vi "ENAmeas.vi"(4 "Error In (no error)":errorcluster, 5 "Meas":T1, 6 "ENA Config":T2={"Sweep Type"=0, "Sweep Mode"=0, "Sweep Points"=201, "Average count"=16, "IF Bandwidth (Hz)"=100000.0, "Power Level (dBm)"=0.0, "Center Freq (Hz)"=0.0, "Span Freq (Hz)"=0.0, "Electrical Delay (s)"=0.0} {"Electrical Delay (s)" format="%.2p"; "Span Freq (Hz)" format="%.2p"; "Center Freq (Hz)" format="%.2p"; "Power Level (dBm)" format="%^.2g"; "IF Bandwidth (Hz)" format="%.1p"; "Sweep Mode" items=["Stepped", "Swept", "Fast Stepped Mode", "Fast Swept Mode"]; "Sweep Type" items=["Linear Sweep", "Logarithmic Sweep", "Segment Sweep", "Power Sweep", "DC Bias"]}, 7 "VISA session":refnum<visa-resource-name>) -> (0 "Error Out":errorcluster, 1 "ENAfreq":dbl[](array[numeric]), 2 "ENAdata":dbl[][](array[numeric]), 3 "dup VISA session":refnum<visa-resource-name>)   [LabVIEW 2017]
uses:
  <instrlib>/Agilent ENA Series/Agilent ENA Series.lvlib
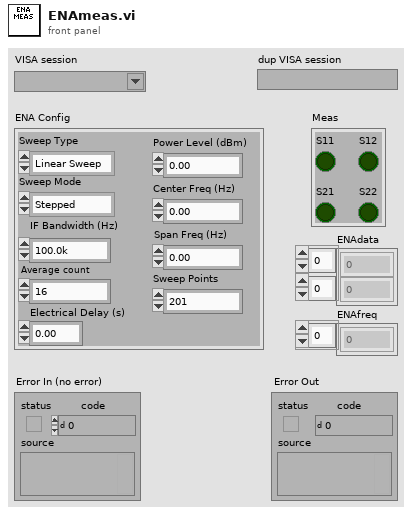
[diagram p1: front panel]
types:
  T1 = cluster{"S11":bool, "S12":bool, "S21":bool, "S22":bool}
  T2 = cluster{"Sweep Type":u16, "Sweep Mode":u16, "Sweep Points":i32, "Average count":i32, "IF Bandwidth (Hz)":dbl, "Power Level (dBm)":dbl, "Center Freq (Hz)":dbl, "Span Freq (Hz)":dbl, "Electrical Delay (s)":dbl}
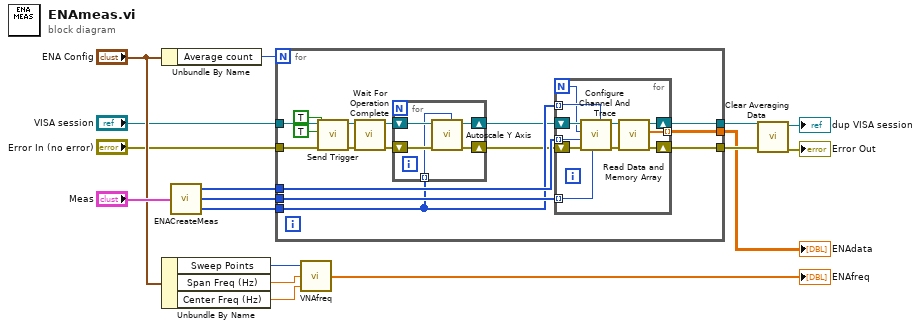
[diagram p0: block diagram]
diagram:
  n1 = Unbundle By Name("ENA Config") -> ("Average count"=w17:i32)
  n2 = Unbundle By Name("ENA Config") -> ("Sweep Points"=w11:i32, "Span Freq (Hz)"=w10:dbl, "Center Freq (Hz)"=w9:dbl)
  n3 = call "ENACreateMeas.vi"("Meas in"="Meas") -> ("Meas parameters"=w15:u16[], "Data format"=w14:u16[], "Active trace"=w13:i32[])
  n4 = for {
    N: w17 -> [_]
    tunnel: [w33] -> w4
    tunnel: "VISA session" -> [w30]
    tunnel: [w32] -> w6
    tunnel: [w31] -> w5
    tunnel: w13 -> [w23]
    tunnel: w15 -> [w25]
    tunnel: w14 -> [w24]
    tunnel: "Error In (no error)" -> [w19]
    n5 = call <instrlib>:"Send Trigger.vi"("error in (no error)"=w19, "Wait for OPC (F: Do not Wait)"=TRUE, "Ignore Trigger Source (F: Do not Ignore)"=TRUE, "VISA resource name"=w30) -> ("error out"=w28:errorcluster, "VISA resource name out"=w29:refnum<visa-resource-name>)  [unwired: 6 in]
    n6 = call <instrlib>:"Wait For Operation Complete.vi"("error in (no error)"=w28, "VISA resource name"=w29) -> ("error out"=w27:errorcluster, "VISA resource name out"=w26:refnum<visa-resource-name>)  [unwired: 8 in]
    n7 = for {
      shift-right: [w36] -> w18
      shift-left: w27 -> [w35]
      shift-right: [w37] -> w22
      shift-left: w26 -> [w38]
      tunnel: w23 -> [w34] mode=indexing
      n8 = call <instrlib>:"Autoscale Y Axis.vi"("Trace (1)"=w34, "error in (no error)"=w35, "VISA resource name"=w38) -> ("error out"=w36:errorcluster, "VISA resource name out"=w37:refnum<visa-resource-name>)  [unwired: 7 in]
    }
    n9 = for {
      N -> [w40]
      shift-right: [w49] -> w31
      shift-left: w22 -> [w47]
      shift-right: [w48] -> w32
      shift-left: w18 -> [w44]
      tunnel: [w39] -> w33 mode=indexing
      tunnel: w25 -> [w43] mode=indexing
      tunnel: w24 -> [w42] mode=indexing
      tunnel: w23 -> [w41] mode=indexing
      n10 = call <instrlib>:"Configure Channel And Trace.vi"("Active Trace (1)"=w41, "Data Format (0: Logarithmic Magnitude)"=w42, "error in (no error)"=w44, "Measurement Parameters (0: S11)"=w43, "Number of Traces (1)"=w40, "VISA resource name"=w47) -> ("error out"=w45:errorcluster, "VISA resource name out"=w46:refnum<visa-resource-name>)  [unwired: 4 in]
      n11 = call <instrlib>:"Read Data and Memory Array.vi"("error in (no error)"=w45, "VISA resource name"=w46) -> ("error out"=w48:errorcluster, "Primary / Real"=w39:dbl[], "VISA resource name out"=w49:refnum<visa-resource-name>)  [unwired: 6 in, 1 out]
    }
  }
  "ENAdata" <- w4
  n12 = call "VNAfreq.vi"("Center Freq (Hz)"=w9, "Span Freq (Hz)"=w10, "Sweep Points"=w11) -> ("VNA Freq"=→"ENAfreq":dbl[])
  n13 = call <instrlib>:"Clear Averaging Data.vi"("error in (no error)"=w6, "VISA resource name"=w5) -> ("error out"=→"Error Out":errorcluster, "VISA resource name out"=→"dup VISA session":refnum<visa-resource-name>)  [unwired: 8 in]
